vi "parse_read_data_string.vi"(8 "error in":errorcluster, 11 "Read Data String":string) -> (0 "error out":errorcluster, 3 "Read Data Cluster":T1)   [LabVIEW 2025, in "Newtons4thEkg.lvlib"]
uses:
  Newtons4thEkg.lvlib
  Typedefs/ReadData.ctl
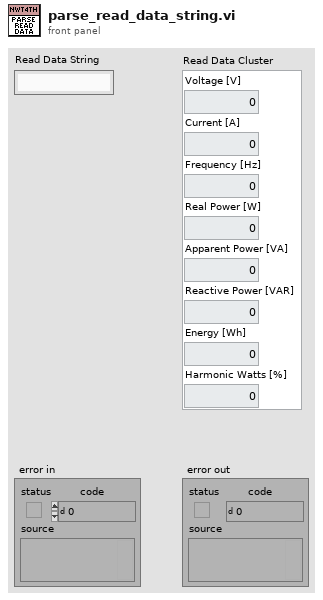
[diagram p1: front panel]
types:
  T1 = typedef "Newtons4thEkg.lvlib/ReadData.ctl" = cluster{"Voltage [V]":dbl, "Current [A]":dbl, "Frequency [Hz]":dbl, "Real Power [W]":dbl, "Apparent Power [VA]":dbl, "Reactive Power [VAR]":dbl, "Energy [Wh]":dbl, "Harmonic Watts [%]":dbl}
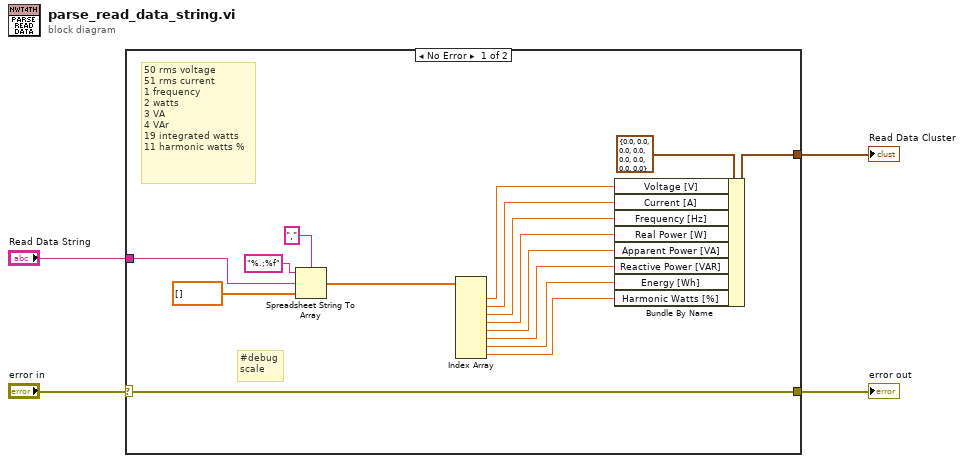
[diagram p0: block diagram]
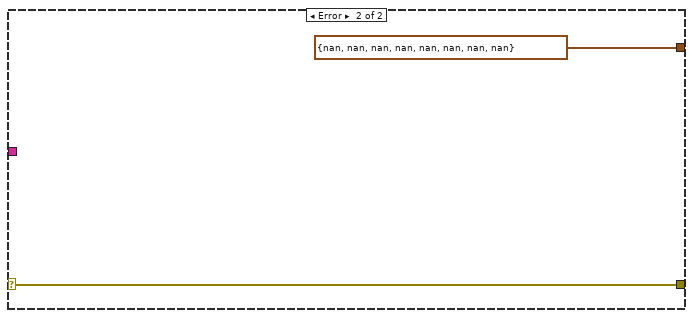
[diagram p2: hidden frame]
diagram:
  n1 = case shown="No Error" "error in" {
    selector: "error in" -> [w6 w21]
    tunnel: [w16 T1 {"Voltage [V]"=nan, "Current [A]"=nan, "Frequency [Hz]"=nan, "Real Power [W]"=nan, "Apparent Power [VA]"=nan, "Reactive Power [VAR]"=nan, "Energy [Wh]"=nan, "Harmonic Watts [%]"=nan} ("Read Data Cluster")] -> w4
    tunnel: [w6 w21] -> w2
    tunnel: "Read Data String" -> [w5 _]
    frame No Error {
      # "#debug\nscale"
      # "50 rms voltage  \n51 rms current\n1 frequency  \n2 watts  \n3 VA  \n4 VAr\n19 integrated watts\n11 harmonic watts %"
      n2 = Spreadsheet String To Array(delimiter (Tab)=",", format string="%.;%f", spreadsheet string=w5, array type (2D Dbl)=dbl[] []) -> (array=w15:dbl[])
      n3 = Index Array(array=w15) -> (element #1=w9:dbl, element #2=w8:dbl, element #3=w14:dbl, element #4=w13:dbl, element #5=w12:dbl, element #6=w11:dbl, element #7=w10:dbl, element #8=w7:dbl)  [unwired: 8 in]
      n4 = Bundle By Name(cluster=T1 {"Voltage [V]"=0.0, "Current [A]"=0.0, "Frequency [Hz]"=0.0, "Real Power [W]"=0.0, "Apparent Power [VA]"=0.0, "Reactive Power [VAR]"=0.0, "Energy [Wh]"=0.0, "Harmonic Watts [%]"=0.0} ("Results"), "Voltage [V]"=w9, "Current [A]"=w8, "Frequency [Hz]"=w14, "Real Power [W]"=w13, "Apparent Power [VA]"=w12, "Reactive Power [VAR]"=w11, "Energy [Wh]"=w10, "Harmonic Watts [%]"=w7) -> (w16:T1)
    }
    frame Error {
    }
  }
  "Read Data Cluster" <- w4
  "error out" <- w2
